vi "PQ Example SELECT.vi"() -> ()   [LabVIEW 2015]
uses:
  Result/PQ Result.lvclass/PQ Result.ctl
  Result/Write Next Row (First Column).vi
  Connection/Execute Command (Result).vi
  Result/Get Column String.vi
  Result/Get Column DBL.vi
  Connection/PQ Connection.lvclass
  Result/PQ Result.lvclass
panel:
  out "error out":errorcluster
  out "Array":T1(array[cluster]) {"Get:Get DBL" format="%#_16g"}
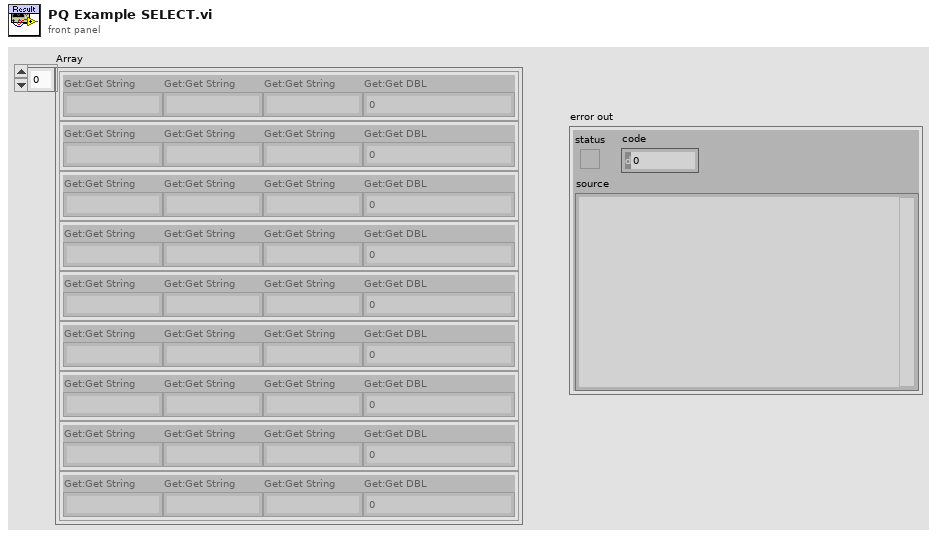
[diagram p1: front panel]
types:
  T1 = cluster{"Get:Get String":string, "Get:Get String":string, "Get:Get String":string, "Get:Get DBL":dbl}[]
  T2 = cluster{"Get:Get String":string, "Get:Get String":string, "Get:Get String":string, "Get:Get DBL":dbl}
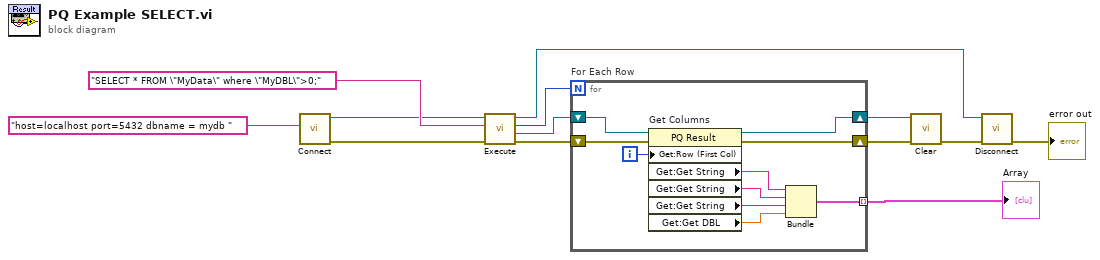
[diagram p0: block diagram]
diagram:
  n1 = call "Connect.vi"("conninfo"="host=localhost port=5432 dbname = mydb ") -> ("error out"=w8:errorcluster, "PQ Connection out"=w10:refnum<class "PQ Connection.lvclass">)  [unwired: 9 in]
  n2 = call-poly "Execute.vi"("error in (no error)"=w8, "SQL (Single Command)"="SELECT * FROM \"MyData\" where \"MyDBL\">0;" ("command"), "PQ Connection in"=w10) -> ("error out"=w2:errorcluster, "First Result with Rows returned"=w4:refnum<class "PQ Result.lvclass">, "Number of Rows"=w3:i32, "PQ Connection out"=w9:refnum<class "PQ Connection.lvclass">)  [unwired: 5 in]
  n3 = for "For Each Row" {
    N: w3 -> [_]
    shift-right: [w23] -> w6
    shift-left: w4 -> [w16]
    shift-right: [w22] -> w1
    shift-left: w2 -> [w15]
    tunnel: [w17] -> w5 mode=indexing
    i -> [w14]
    n4 = property on="Get Columns" class="PQ Result"(reference=w16, error in=w15, "Get:Row (First Col)"=w14) -> (reference out=w23:refnum<class "PQ Result.lvclass">, error out=w22:errorcluster, "Get:Get String"=w21:string, "Get:Get String"=w20:string, "Get:Get String"=w19:string, "Get:Get DBL"=w18:dbl)
    n5 = Bundle("Get:Get String"=w21, "Get:Get String"=w20, "Get:Get String"=w19, "Get:Get DBL"=w18) -> (w17:T2)  [unwired: 1 in]
  }
  "Array" <- w5
  n6 = call "Clear.vi"("error in (no error)"=w1, "PQ Result  in"=w6) -> ("error out"=w11:errorcluster)  [unwired: 9 in]
  n7 = call "Disconnect.vi"("error in (no error)"=w11, "PQ Connection in"=w9) -> ("error out"=→"error out":errorcluster)  [unwired: 9 in]
